vi "Convert Array  (SubVI)V2.0.vi"() -> (0 "Conversion Array":dbl[](array[numeric]))   [LabVIEW 2012]
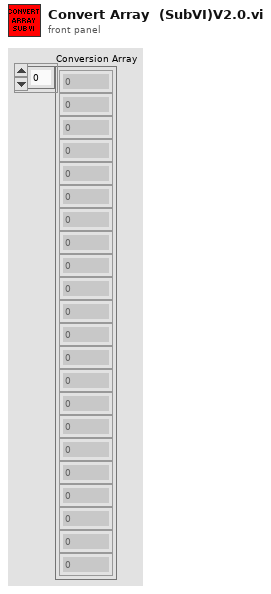
[diagram p1: front panel]
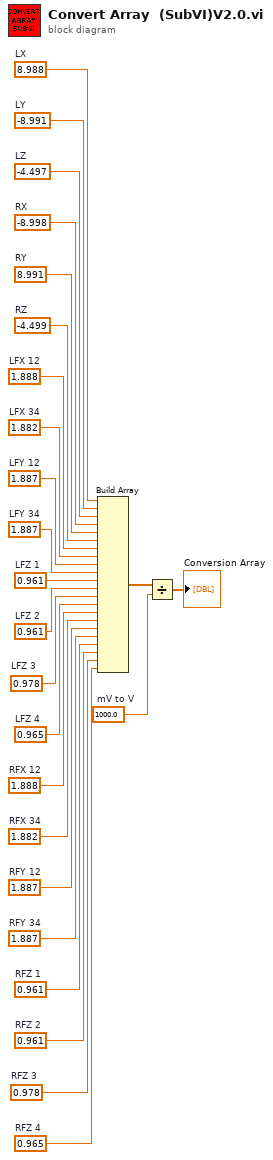
[diagram p0: block diagram]
diagram:
  w3 = 1000.0  # mV to V
  w23 = 0.961  # RFZ 2
  w22 = 0.961  # RFZ 1
  w24 = 0.978  # RFZ 3
  w25 = 0.965  # RFZ 4
  w18 = 1.888  # RFX 12
  w19 = 1.882  # RFX 34
  w20 = 1.887  # RFY 12
  w21 = 1.887  # RFY 34
  w7 = -8.998  # RX
  w6 = -4.497  # LZ
  w8 = 8.991  # RY
  w9 = -4.499  # RZ
  w4 = 8.988  # LX
  w5 = -8.991  # LY
  w15 = 0.961  # LFZ 2
  w14 = 0.961  # LFZ 1
  w16 = 0.978  # LFZ 3
  w17 = 0.965  # LFZ 4
  w10 = 1.888  # LFX 12
  w11 = 1.882  # LFX 34
  w12 = 1.887  # LFY 12
  w13 = 1.887  # LFY 34
  n1 = Build Array(w4, w5, w6, w7, w8, w9, w10, w11, w12, w13, w14, w15, w16, w17, w18, w19, w20, w21, w22, w23, w24, w25) -> (w2:dbl[])
  n2 = Divide(x=w2, y=w3) -> (x/y=→"Conversion Array":dbl[])
